vi "Test_freq_generator_5782.vi"() -> ()   [LabVIEW 2013]
uses:
  <vilib>/measure/maspectr.llb/Power Spectrum and PSD Export Mode.ctl
  <vilib>/measure/maspectr.llb/FFT Power Spectrum and PSD for 1 Chan (CDB).vi
  <vilib>/measure/NI_MAPro.lvlib
panel:
  out "power spectrum":cluster{"f0":dbl, "df":dbl, "magnitude":dbl[]}(graph)
  out "Cos":fxp<+/-,16,0>[][](array[numeric])
  out "simdata":i16[][](array[numeric])
  out "Sin":fxp<+/-,16,0>[][](array[numeric])
  out "Waveform Graph 2":i16[](graph)
  out "Waveform Graph":dbl[][](graph)
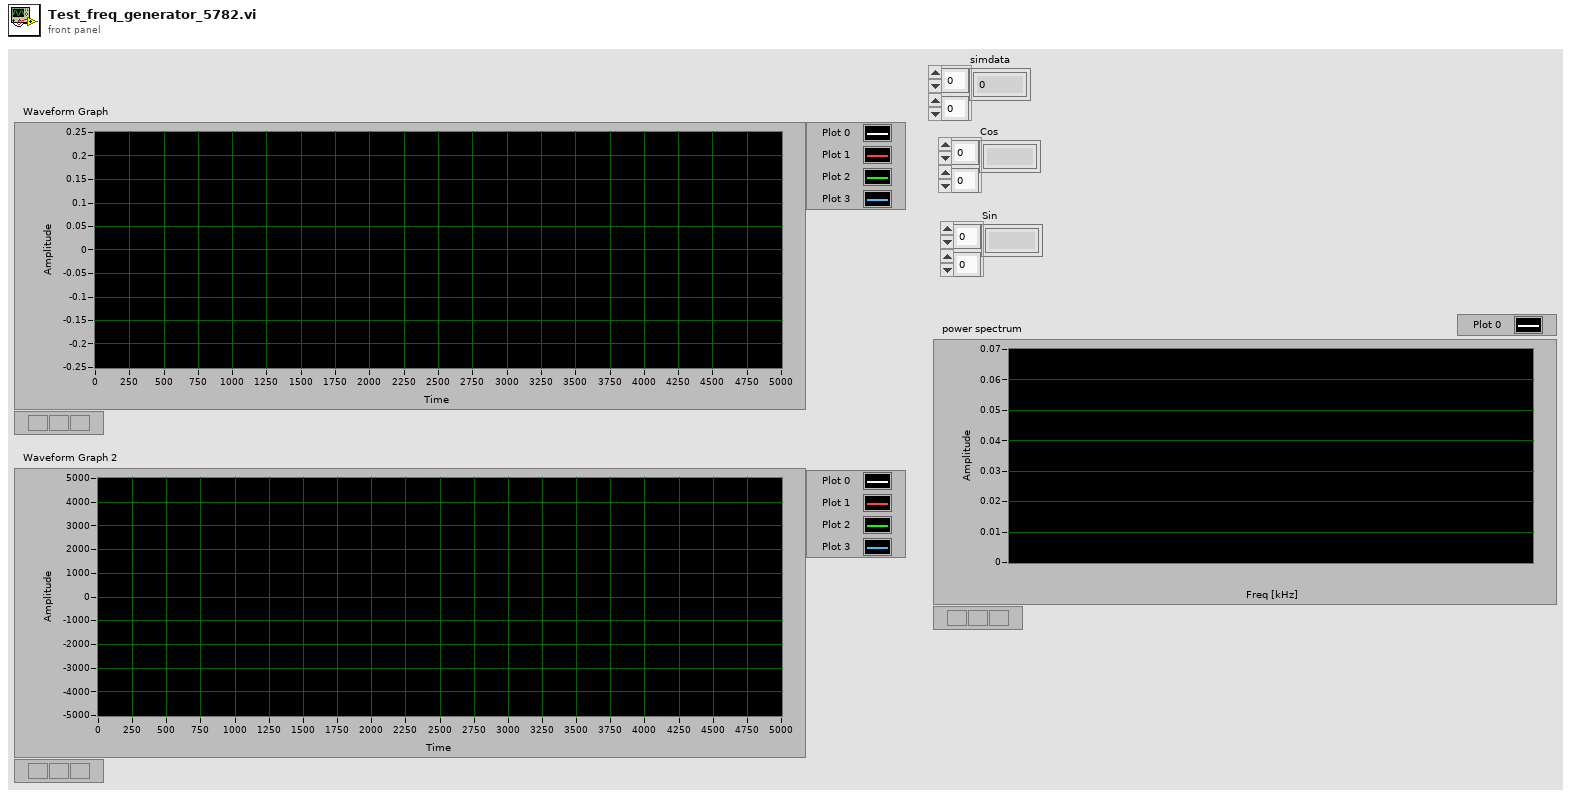
[diagram p1: front panel]
types:
  T1 = typedef "NI_MAPro.lvlib/Power Spectrum and PSD Export Mode.ctl" = u16
  T2 = typedef "I16 array size 2.ctl" = i16[]
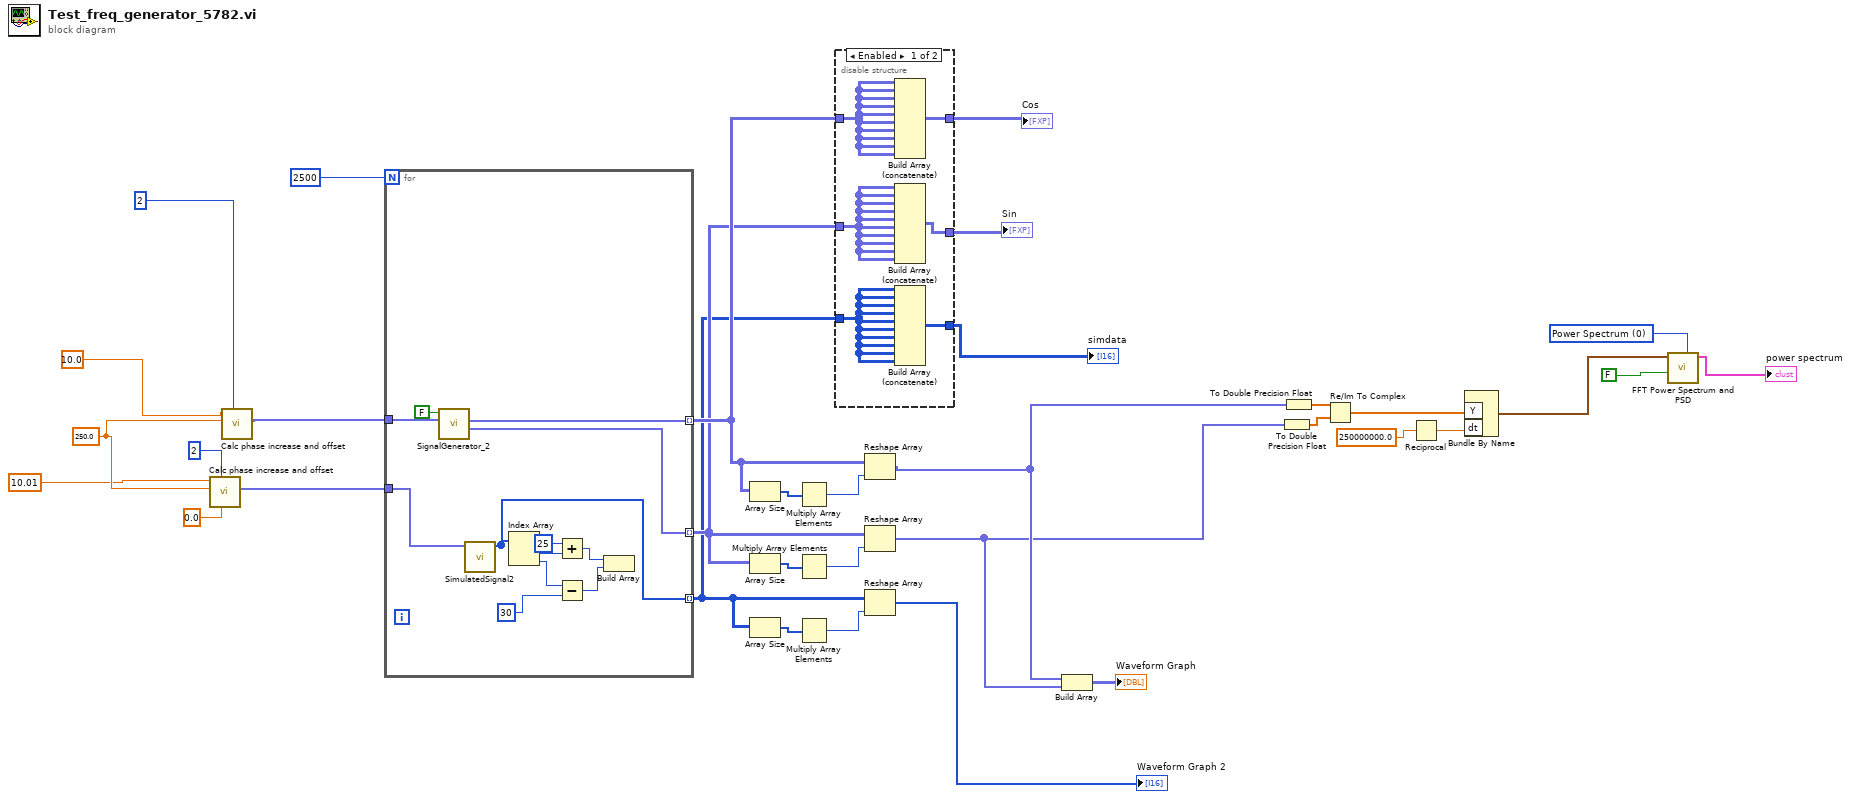
[diagram p0: block diagram]
diagram:
  w21 = T1 0 items=["Power Spectrum", "Power Spectral Density"] ("export mode")
  w33 = 250.0 ("fclk (800MHz)")
  n1 = call "Calc phase increase and offset.vi"("Phase offset (deg)"=0.0, "# of DDS"=2, "fclk (MHz)"=w33, "f_generated (MHz)"=10.01) -> ("Phase out"=w23:fxp<+,64,64>[])  [unwired: 5 in, 2 out]
  n2 = call "Calc phase increase and offset.vi"("# of DDS"=2, "fclk (MHz)"=w33, "f_generated (MHz)"=10.0) -> ("Phase out"=w24:fxp<+,64,64>[])  [unwired: 6 in, 2 out]
  n3 = for {
    N: 2500 -> [_]
    tunnel: w24 -> [w46]
    tunnel: [w45] -> w8 mode=indexing
    tunnel: w23 -> [w44]
    tunnel: [w35] -> w4 mode=indexing
    tunnel: [w42] -> w5 mode=indexing
    n4 = call "SignalGenerator_2.vi"("Phase"=w46, "reset"=FALSE) -> ("Sine out"=w42:fxp<+/-,16,0>[], "Cosine out"=w45:fxp<+/-,16,0>[])  [unwired: 8 in]
    n5 = call "SimulatedSignal2.vi"("Phase"=w44) -> ("output"=w35:T2)  [unwired: 9 in, 1 out]
    n6 = Index Array(array=w35) -> (element #1=w41:i16, element #2=w39:i16)  [unwired: 2 in]
    n7 = Add(x=i16 25, y=w41) -> (x+y=w37:i16)
    n8 = Subtract(x=w39, y=i16 30 ("x")) -> (x-y=w36:i16)
    n9 = Build Array(w37, w36) -> ()  [unwired: 1 out]
  }
  n10 = Array Size(array=w8) -> (size(s)=w28:i32[])
  n11 = Array Size(array=w5) -> (size(s)=w10:i32[])
  n12 = Array Size(array=w4) -> (size(s)=w25:i32[])
  n13 = Multiply Array Elements(1:w28) -> (0:w27:i32)
  n14 = Multiply Array Elements(1:w10) -> (0:w11:i32)
  n15 = Multiply Array Elements(1:w25) -> (0:w26:i32)
  n16 = disable-structure shown="Enabled" {
    disable-tunnel: w5 -> [w52 w54]
    disable-tunnel: [w51 w55] -> w7
    disable-tunnel: [w50 w54] -> w6
    disable-tunnel: w8 -> [w49 w55]
    disable-tunnel: w4 -> [w48 w53]
    disable-tunnel: [w47 w53] -> w3
    frame Enabled {
      n17 = Build Array (concatenate)(w49, w49, w49, w49, w49, w49, w49, w49, w49, w49) -> (w51:fxp<+/-,16,0>[][])
      n18 = Build Array (concatenate)(w52, w52, w52, w52, w52, w52, w52, w52, w52, w52) -> (w50:fxp<+/-,16,0>[][])
      n19 = Build Array (concatenate)(w48, w48, w48, w48, w48, w48, w48, w48, w48, w48) -> (w47:i16[][])
    }
    frame Disabled {
    }
  }
  "Sin" <- w6
  "simdata" <- w3
  "Cos" <- w7
  n20 = Reshape Array(w8, w27) -> (w2:fxp<+/-,16,0>[])
  n21 = Reshape Array(w5, w11) -> (w1:fxp<+/-,16,0>[])
  n22 = Reshape Array(w4, w26) -> (→"Waveform Graph 2":i16[])
  n23 = Build Array(w2, w1) -> (→"Waveform Graph":fxp<+/-,16,0>[][])
  n24 = To Double Precision Float(number=w1) -> (double precision float=w14:dbl[])
  n25 = To Double Precision Float(number=w2) -> (double precision float=w15:dbl[])
  n26 = Re/Im To Complex(1:w14, 2:w15) -> (0:w13:cdb[])
  n27 = Reciprocal(x=250000000.0 ("dt")) -> (1/x=w17:dbl)
  n28 = Bundle By Name("Y"=w13, "dt"=w17) -> (w20:waveform(cdb))  [unwired: 1 in]
  n29 = call-poly <vilib>:"FFT Power Spectrum and PSD.vi"("export mode"=w21, "dB On (F)"=FALSE, "time signal"=w20) -> ("Power Spectrum / PSD"=→"power spectrum":cluster{"f0":dbl, "df":dbl, "magnitude":dbl[]})  [unwired: 5 in, 3 out]
